vi "33522A_control.vi"   [LabVIEW 2019]
uses:
  <userlib>/_TI-LA/Instr Drivers/Signal Generator/33XXX/Driver/Base/Agilent 33XXX Series.lvlib
  <userlib>/_TI-LA/Instr Drivers/Signal Generator/3352x/Driver/Base/Agilent 3352X Series.lvlib
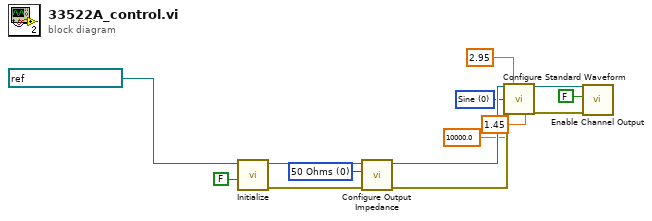
[diagram p0: block diagram]
diagram:
  w5 = 0 items=["Sine"=0, "Square"=1, "Ramp"=2, "Noise"=3, "DC"=4, "Triangle"=5, "Pulse"=6, "Sinc"=11, "D-Lorentz"=12, "Gaussian"=13, "Expo Fall"=14, "Expo Rise"=15, "Haversine"=16] ("Waveform Function (0: Sine)")
  w6 = u16 0 items=["50 Ohms", "High Impedance", "User Defined"] ("Impedance (0: 50 Ohms)")
  n1 = call <userlib>:"Initialize.vi"("Reset (Enable)"=FALSE, "VISA resource name"=refnum<visa-resource-name> "GPIB0::11::INSTR") -> ("error out"=w14:errorcluster, "VISA resource name out"=w13:refnum<visa-resource-name>)  [unwired: 8 in]
  n2 = call <userlib>:"Configure Output Impedance.vi"("error in (no error)"=w14, "Impedance (0: 50 Ohms)"=w6, "VISA resource name"=w13) -> ("error out"=w11:errorcluster, "VISA resource name out"=w12:refnum<visa-resource-name>)  [unwired: 7 in]
  n3 = call <userlib>:"Configure Standard Waveform.vi"("VISA resource name"=w12, "Amplitude (0.1 Vpp)"=2.95, "Waveform Function (0: Sine)"=w5, "Frequency/Sample Rate/Bandwidth (1000 Hz)"=10000.0, "error in (no error)"=w11, "DC Offset (0 V)"=1.45) -> ("VISA resource name out"=w10:refnum<visa-resource-name>, "error out"=w9:errorcluster)  [unwired: 8 in]
  n4 = call <userlib>:"Enable Channel Output.vi"("error in (no error)"=w9, "Enable Output (T: Enable)"=FALSE, "VISA resource name"=w10) -> ()  [unwired: 7 in, 2 out]
